vi "Annotate Poles.vi"(1 "Column Data":T2, 2 "Spacing":dbl, 3 "Image In":T1) -> (0 "Image Out":T1)   [LabVIEW 2013]
doc: "Draw green rectangles around the particles identified to be a pole."
uses:
  Gridded Particles.ctl
  <vilib>/vision/Image Controls.llb/IMAQ Image.ctl
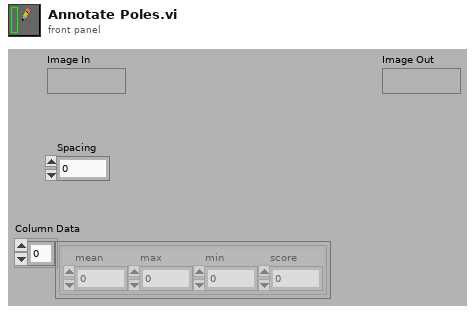
[diagram p1: front panel]
types:
  T1 = typedef "IMAQ Image.ctl" = refnum<image>
  T2 = typedef "Gridded Particles.ctl" = cluster{"mean":dbl, "max":dbl, "min":dbl, "score":dbl}[]
  T3 = cluster{"Spacing":dbl, "Top":i32, dbl, "Bottom":i32}
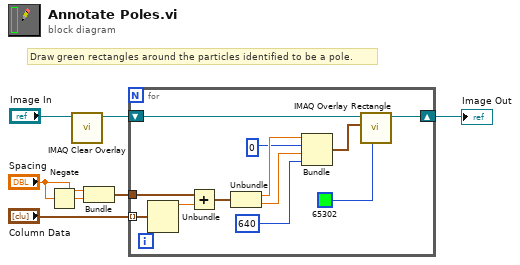
[diagram p0: block diagram]
diagram:
  # "Draw green rectangles around the particles identified to be a pole."
  n1 = Negate(x="Spacing") -> (-x=w3:dbl)
  n2 = call "IMAQ Clear Overlay"("Image"="Image In") -> ("Image Out"=w6:T1)  [unwired: 2 in, 8 out]
  n3 = Bundle("Spacing"="Spacing", w3) -> (w1:cluster{"Spacing":dbl, dbl})  [unwired: 1 out]
  n4 = for {
    shift-right: [w8] -> w5
    shift-left: w6 -> [w16]
    tunnel: "Column Data" -> [w19] mode=indexing
    tunnel: w1 -> [w18]
    n5 = Unbundle(w19) -> ("mean"=w15:dbl)  [unwired: 3 out]
    n6 = Add(x=w18, y=w15) -> (x+y=w14:cluster{"Spacing":dbl, dbl})
    n7 = Unbundle(w14) -> ("Spacing"=w13:dbl, w12:dbl)
    n8 = Bundle("Spacing"=w13, "Top"=0, w12, "Bottom"=640) -> (w9:T3)  [unwired: 1 out]
    n9 = call "IMAQ Overlay Rectangle"("Color"=u32 65302, "Rectangle"=w9, "Image"=w16) -> ("Image Out"=w8:T1)  [unwired: 3 in, 5 out]
  }
  "Image Out" <- w5
